vi "Acquire Data from Hardware.vi"(8 "error in (no error)":errorcluster, 11 "Hardware Configuration":T1) -> (0 "error out":errorcluster, 2 "Graph Data":waveform(dbl)[](array[waveform]))   [LabVIEW 2019]
doc: "Generates sample waveforms according to the signal type in the HW Config input."
uses:
  controls/HW Configuration.ctl
  controls/Simulated Signal Type.ctl
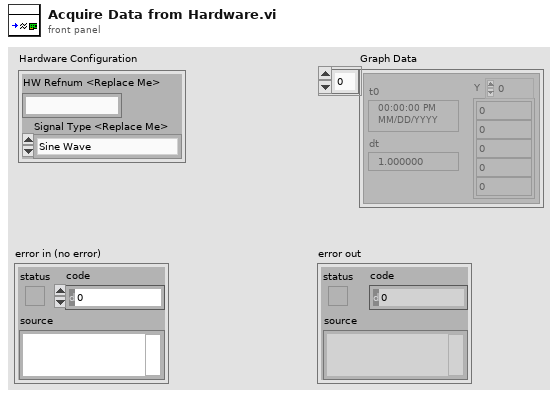
[diagram p1: front panel]
types:
  T1 = typedef "HW Configuration.ctl" = cluster{"HW Refnum <Replace Me>":string, "Signal Type <Replace Me>":T2}
  T2 = typedef "Simulated Signal Type.ctl" = enum16{"Sine Wave", "Square Wave"}
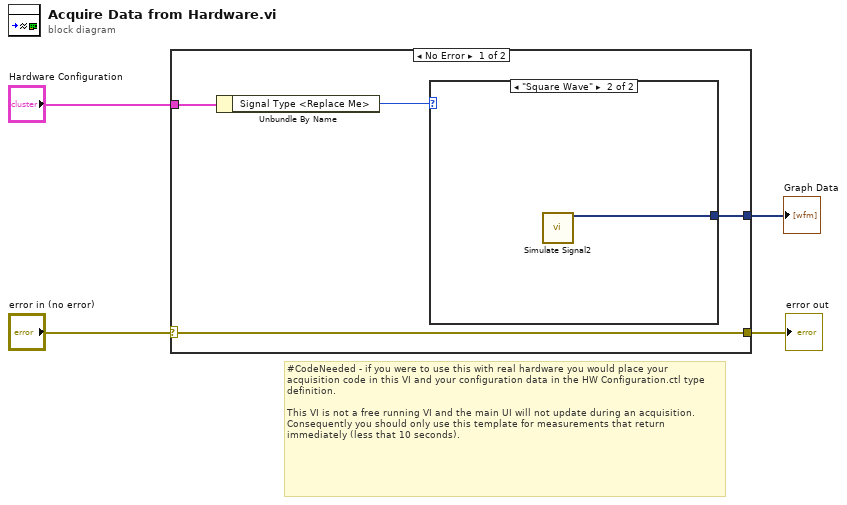
[diagram p0: block diagram]
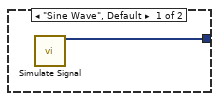
[diagram p2: hidden frame]
diagram:
  # "#CodeNeeded - if you were to use this with real hardware you would place your acquisition code in this VI and your configuration data in the HW Configuration.ctl type definition.\n\nThis VI is not a free running VI and the main UI will not update during an acquisition.  Consequently you should only use this template for measurements that return immediately (less that 10 seconds)."
  n1 = case shown="No Error" "error in (no error)" {
    selector: "error in (no error)" -> [w8 w11]
    tunnel: [w8 w11] -> w3
    tunnel: "Hardware Configuration" -> [w7 _]
    tunnel: [w6 _] -> w1
    frame No Error {
      n2 = Unbundle By Name(w7) -> ("Signal Type <Replace Me>"=w5:T2)
      n3 = case shown="\"Square Wave\"" w5 {
        tunnel: [w9 w10] -> w6
        frame "Sine Wave", Default {
          n4 = call "Simulate Signal"() -> ("Sine"=w9:dynamicdata)  [unwired: 14 in, 1 out]
        }
        frame "Square Wave" {
          n5 = call "Simulate Signal2"() -> ("Square"=w10:dynamicdata)  [unwired: 14 in, 1 out]
        }
      }
    }
    frame Error {
    }
  }
  "error out" <- w3
  "Graph Data" <- w1
